vi "TriggerSpectraWizAcquire.vi"(6 "Stage events":refnum<queue>, 8 "error in (no error)":errorcluster, 11 "Microscope in":refnum<class "Microscope.lvclass">) -> (0 "error out":errorcluster, 3 "Microscope out":refnum<class "Microscope.lvclass">)   [LabVIEW 2012, in "Microscope.lvclass"]
uses:
  classes/Microscope.lvclass
  typedefs/StageEvent.ctl
  classes/Microscope.lvclass/Microscope.ctl
  Spectrometer/Events/SpectrometerEvents.ctl
  Spectrometer/SpectrometerSpectraWiz.llb/StellarNet Globals.vi
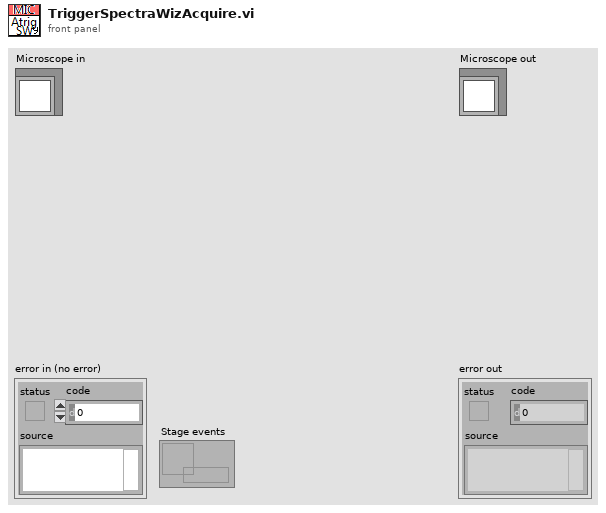
[diagram p1: front panel]
types:
  T1 = typedef "SpectrometerEvents.ctl" = enum16{"TimeOut", "Init Programmatically", "Init Button", "Init Background", "Acquire Background", "Acquire"}
  T2 = typedef "StageEvent.ctl" = enum16{"stage.TimeOut", "stage.FlushData", "stage.GetPosition", "stage.Init", "stage.MoveTo1", "stage.MoveTo2", "stage.MoveTo3", "stage.Stop"}
  T3 = typedef "ScanMode.ctl" = enum16{"None", "Continuous", "Point Scan (CH3 cursor)", "Point Scan Move (CH3 cursor)", "Grab", "Grab Move Stage", "Grab Move Z-stage", "Cont. Move Z-stage", "Spec Move Stage", "Spec Move Cont", "Surf Calib"}
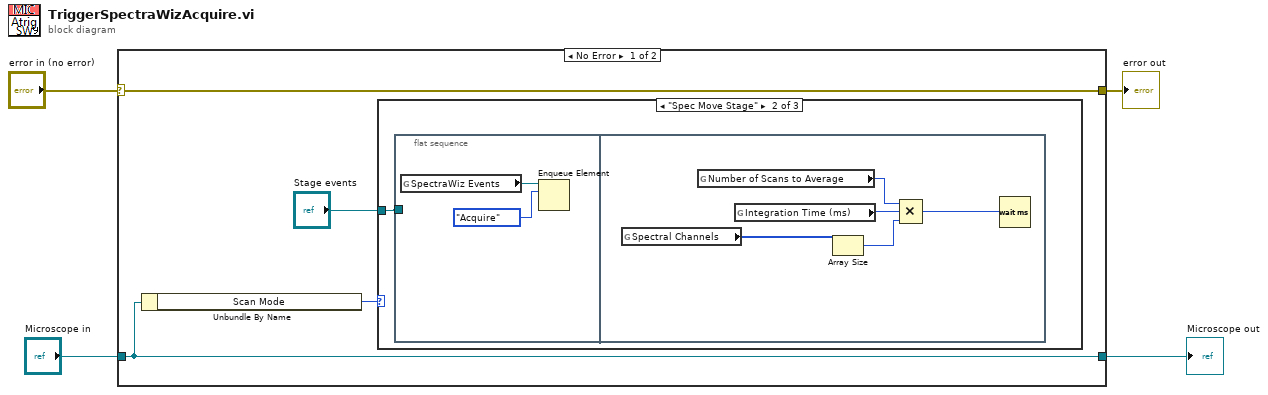
[diagram p0: block diagram]
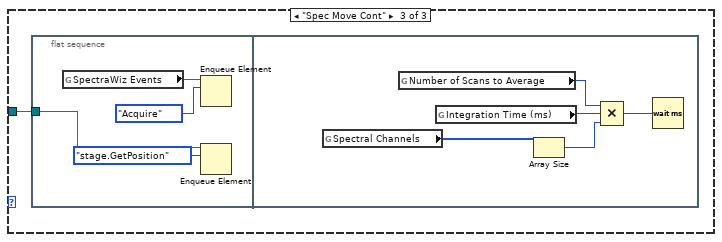
[diagram p3: hidden frame]
diagram:
  n1 = case shown="No Error" "error in (no error)" {
    selector: "error in (no error)" -> [w8 w28]
    tunnel: [w8 w28] -> w3
    tunnel: [w7 w27] -> w1
    tunnel: "Microscope in" -> [w7 w27]
    frame No Error {
      n2 = Unbundle By Name(w7) -> ("Scan Mode"=w6:T3)
      n3 = case shown="\"Spec Move Stage\"" w6 {
        tunnel: "Stage events" -> [_ w9 w17]
        frame "None", Default {
        }
        frame "Spec Move Stage" {
          n4 = flat-sequence {
            tunnel: w9 -> [_]
            frame #0 {
              n5 = global read "StellarNet Globals.vi" "SpectraWiz Events"() -> (w11:refnum<queue>)
              n6 = Enqueue Element(queue=w11, element=SpectrometerEvents."Acquire") -> ()  [unwired: 2 in, 3 out]
            }
            frame #1 {
              n7 = global read "StellarNet Globals.vi" "Spectral Channels"() -> (w12:i32[])
              n8 = global read "StellarNet Globals.vi" "Number of Scans to Average"() -> (w14:i32)
              n9 = global read "StellarNet Globals.vi" "Integration Time (ms)"() -> (w15:i32)
              n10 = Array Size(array=w12) -> (size(s)=w13:i32)
              n11 = Compound Arithmetic op=MULTIPLY(w14, w15, w13) -> (w16:i32)
              n12 = Wait (ms)(milliseconds to wait=w16) -> ()  [unwired: 1 out]
            }
          }
        }
        frame "Spec Move Cont" {
          n13 = flat-sequence {
            tunnel: w17 -> [w19]
            frame #0 {
              n14 = global read "StellarNet Globals.vi" "SpectraWiz Events"() -> (w21:refnum<queue>)
              n15 = Enqueue Element(queue=w21, element=SpectrometerEvents."Acquire") -> ()  [unwired: 2 in, 3 out]
              n16 = Enqueue Element(queue=w19, element=StageEvent."stage.GetPosition") -> ()  [unwired: 2 in, 3 out]
            }
            frame #1 {
              n17 = global read "StellarNet Globals.vi" "Spectral Channels"() -> (w23:i32[])
              n18 = global read "StellarNet Globals.vi" "Number of Scans to Average"() -> (w25:i32)
              n19 = global read "StellarNet Globals.vi" "Integration Time (ms)"() -> (w26:i32)
              n20 = Array Size(array=w23) -> (size(s)=w24:i32)
              n21 = Compound Arithmetic op=MULTIPLY(w25, w26, w24) -> (w22:i32)
              n22 = Wait (ms)(milliseconds to wait=w22) -> ()  [unwired: 1 out]
            }
          }
        }
      }
    }
    frame Error {
    }
  }
  "error out" <- w3
  "Microscope out" <- w1
